vi "应变器转换.vi"() -> ()   [LabVIEW 2018]
uses:
  <vilib>/Utility/TradDaqScaling.llb/Convert Strain Gauge Reading (scaler).vi
panel:
  in  "Vinit (0.0)":sgl format="%0.6f"
  in  "v (0.0)":sgl format="%0.6f"
  in  "GF (2.0)":sgl=2.0 format="%0.6f"
  in  "Rg (120)":sgl=120.0 format="%0.6f"
  in  "停止":bool
  out "仪表":dbl(knob) scale=-1.0..1.0
  in  "Rl (0.0)":sgl format="%0.6f"
  in  "Vex (3.33)":sgl=3.33 format="%0.6f"
  in  "应变计电压":dbl
  in  "Bridge Configuration\n(3:Half Bridge II)":u16(ring)=3 caption="电桥配置\n（3：半桥II）" items=["四分之一电桥 I", "四分之一电桥 II", "半桥 I", "半桥 II", "全桥 I", "全桥 II", "全桥 III"]
  out "字符串":string="转换应变器读数"
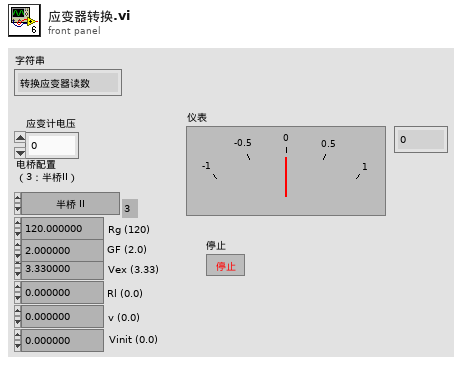
[diagram p1: front panel]
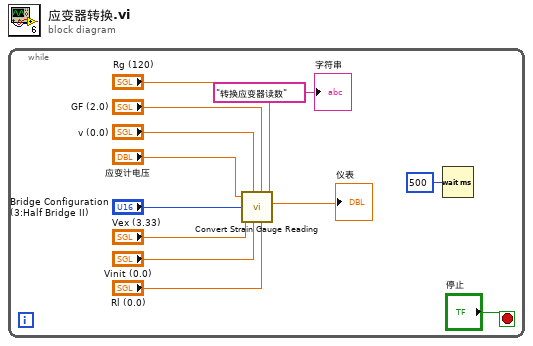
[diagram p0: block diagram]
diagram:
  n1 = while {
    stop <- "停止" stop-if-true
    n2 = call-poly <vilib>:"Convert Strain Gauge Reading.vi"("Vsg (0.0)"="应变计电压", "v (0.0)"="v (0.0)", "Bridge Configuration\n(3:Half Bridge II)"="Bridge Configuration\n(3:Half Bridge II)", "Vex (3.33)"="Vex (3.33)", "Vinit (0.0)"="Vinit (0.0)", "GF (2.0)"="GF (2.0)", "Rg (120)"="Rg (120)", "Rl (0.0)"="Rl (0.0)") -> ("Strain"=→"仪表":sgl)  [unwired: 2 in]
    n3 = Wait (ms)(milliseconds to wait=u32 500 ("等待时间（毫秒）")) -> ()  [unwired: 1 out]
    "字符串" <- "转换应变器读数"
  }
